vi "Bodies_Init_DH2.vi"(8 "error in (no error)":errorcluster, 10 "KnownDHVars":T3(array[cluster]), 11 "Body.lvclass In":refnum<class "Bodies.lvclass">) -> (0 "error out":errorcluster, 3 "Body.lvclass Out":refnum<class "Bodies.lvclass">)   [LabVIEW 2015, in "Bodies.lvclass"]
uses:
  Bodies.lvclass
  DH_parameters.ctl
  PointOnBody.ctl
  <vilib>/Analysis/Matrix/Datatypes/RealMatrix.ctl
  Bodies.lvclass/Bodies.ctl
  <vilib>/gmath/NI_Gmath.lvlib
  <vilib>/Analysis/Matrix/NI_Matrix.lvlib
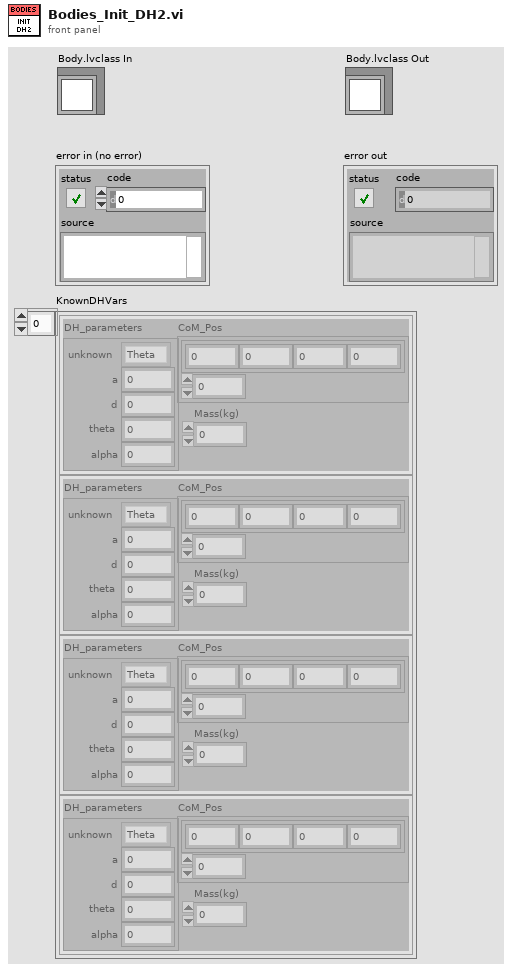
[diagram p1: front panel]
types:
  T1 = typedef "Bodies.lvclass/DH_parameters.ctl" = cluster{"unknown":enum16{"Theta", "Alpha", "a", "d"}, "a":dbl, "d":dbl, "alpha":dbl, "theta":dbl}
  T2 = typedef "Bodies.lvclass/PointOnBody.ctl" = cluster{"Coord4":dbl[], "ID":i32}
  T3 = cluster{"DH_parameters":T1, "CoM_Pos":T2, "Mass(kg)":dbl}[]
  T4 = typedef "NI_Matrix.lvlib/RealMatrix.ctl" = dbl[][]
  T5 = cluster{"Y Values":dbl[][], "Tables":i32[][][], "Variables input decode":i32[], "Variables output decode":i32[]}
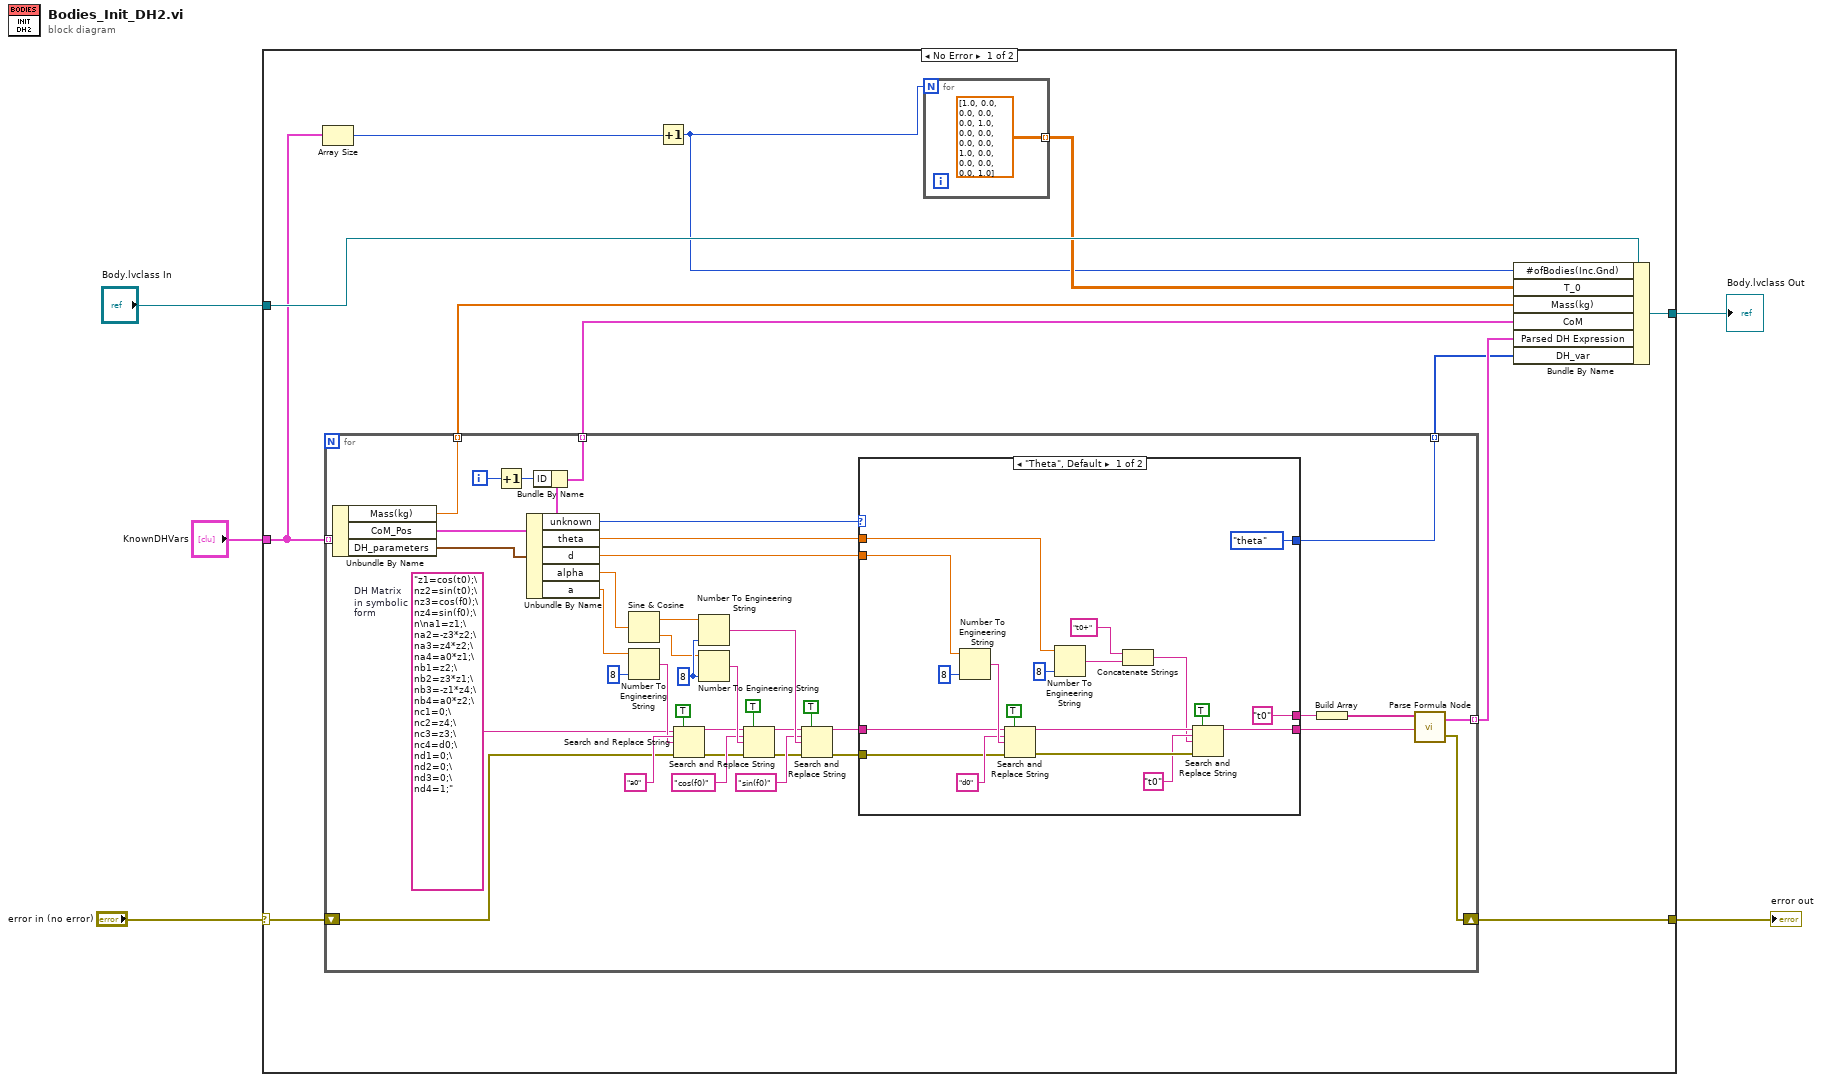
[diagram p0: block diagram]
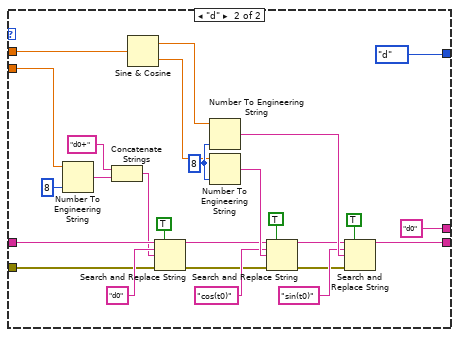
[diagram p2: hidden frame]
diagram:
  n1 = case shown="No Error" "error in (no error)" {
    selector: "error in (no error)" -> [w17 w104]
    tunnel: "KnownDHVars" -> [w11 _]
    tunnel: [w12 w104] -> w5
    tunnel: "Body.lvclass In" -> [w16 w103]
    tunnel: [w14 w103] -> w2
    frame No Error {
      n2 = Array Size(array=w11) -> (size(s)=w10:i32)
      n3 = for {
        tunnel: w11 -> [w55] mode=indexing
        tunnel: [w56] -> w13 mode=indexing
        shift-right: [w57] -> w12
        shift-left: w17 -> [w33]
        tunnel: [w54] -> w8 mode=indexing
        tunnel: [w23] -> w7 mode=indexing
        tunnel: [w20] -> w6 mode=indexing
        i -> [w21]
        w39 = i16 8 ("precision (6)")
        w48 = "z1=cos(t0);\nz2=sin(t0);\nz3=cos(f0);\nz4=sin(f0);\n\na1=z1;\na2=-z3*z2;\na3=z4*z2;\na4=a0*z1;\nb1=z2;\nb2=z3*z1;\nb3=-z1*z4;\nb4=a0*z2;\nc1=0;\nc2=z4;\nc3=z3;\nc4=d0;\nd1=0;\nd2=0;\nd3=0;\nd4=1;"  # DH Matrix in symbolic form
        n4 = Unbundle By Name(w55) -> ("Mass(kg)"=w54:dbl, "CoM_Pos"=w22:T2, "DH_parameters"=w53:T1)
        n5 = Increment(x=w21) -> (x+1=w19:i32)
        n6 = Unbundle By Name(w53) -> ("unknown"=w31:enum16{"Theta", "Alpha", "a", "d"}, "theta"=w30:dbl, "d"=w29:dbl, "alpha"=w36:dbl, "a"=w35:dbl)
        n7 = Bundle By Name(cluster=w22, "ID"=w19) -> (w20:T2)
        n8 = Sine & Cosine(0:w36) -> (1:w37:dbl, 2:w38:dbl)
        n9 = Number To Engineering String(2:i16 8 ("precision (6)"), 4:w35) -> (0:w50:string)  [unwired: 2 in]
        n10 = Search and Replace String(replace all?=TRUE ("replace all? (F)"), input string=w48, search string="a0", replace string=w50, error in=w33) -> (result string=w34:string, error out=w32:errorcluster)  [unwired: 3 in, 2 out]
        n11 = Number To Engineering String(2:w39, 4:w37) -> (0:w46:string)  [unwired: 2 in]
        n12 = Number To Engineering String(2:w39, 4:w38) -> (0:w47:string)  [unwired: 2 in]
        n13 = Search and Replace String(replace all?=TRUE ("replace all? (F)"), input string=w34, search string="cos(f0)", replace string=w47, error in=w32) -> (result string=w42:string, error out=w41:errorcluster)  [unwired: 3 in, 2 out]
        n14 = Search and Replace String(replace all?=TRUE ("replace all? (F)"), input string=w42, search string="sin(f0)", replace string=w46, error in=w41) -> (result string=w28:string, error out=w27:errorcluster)  [unwired: 3 in, 2 out]
        n15 = case shown="\"Theta\", Default" w31 {
          tunnel: w30 -> [w75 w79]
          tunnel: w29 -> [w70 w99]
          tunnel: w28 -> [w69 w98]
          tunnel: w27 -> [w68 w97]
          tunnel: [w60 w78] -> w26
          tunnel: ["t0" ("string") "d0" ("string")] -> w25
          tunnel: [enum16{"theta", "d"}."theta" ("Enum") enum16{"theta", "d"}."d" ("Enum")] -> w23
          frame "Theta", Default {
            n16 = Number To Engineering String(2:i16 8 ("precision (6)"), 4:w70) -> (0:w73:string)  [unwired: 2 in]
            n17 = Search and Replace String(replace all?=TRUE ("replace all? (F)"), input string=w69, search string="d0", replace string=w73, error in=w68) -> (result string=w63:string, error out=w64:errorcluster)  [unwired: 3 in, 2 out]
            n18 = Number To Engineering String(2:i16 8 ("precision (6)"), 4:w75) -> (0:w67:string)  [unwired: 2 in]
            n19 = Concatenate Strings("t0+" ("string"), w67) -> (w61:string)
            n20 = Search and Replace String(replace all?=TRUE ("replace all? (F)"), input string=w63, search string="t0", replace string=w61, error in=w64) -> (result string=w60:string)  [unwired: 3 in, 3 out]
          }
          frame "d" {
            w84 = i16 8 ("precision (6)")
            n21 = Number To Engineering String(2:i16 8 ("precision (6)"), 4:w99) -> (0:w95:string)  [unwired: 2 in]
            n22 = Concatenate Strings("d0+" ("string"), w95) -> (w94:string)
            n23 = Sine & Cosine(0:w79) -> (1:w82:dbl, 2:w83:dbl)
            n24 = Search and Replace String(replace all?=TRUE ("replace all? (F)"), input string=w98, search string="d0", replace string=w94, error in=w97) -> (result string=w81:string, error out=w80:errorcluster)  [unwired: 3 in, 2 out]
            n25 = Number To Engineering String(2:w84, 4:w82) -> (0:w91:string)  [unwired: 2 in]
            n26 = Number To Engineering String(2:w84, 4:w83) -> (0:w92:string)  [unwired: 2 in]
            n27 = Search and Replace String(replace all?=TRUE ("replace all? (F)"), input string=w81, search string="cos(t0)", replace string=w92, error in=w80) -> (result string=w87:string, error out=w86:errorcluster)  [unwired: 3 in, 2 out]
            n28 = Search and Replace String(replace all?=TRUE ("replace all? (F)"), input string=w87, search string="sin(t0)", replace string=w91, error in=w86) -> (result string=w78:string)  [unwired: 3 in, 3 out]
          }
        }
        n29 = Build Array(w25) -> (w24:string[])
        n30 = call <vilib>:"Parse Formula Node.vi"("formula"=w26, "Variables Input"=w24) -> ("error out"=w57:errorcluster, "Parsed Formula Node"=w56:T5)  [unwired: 2 in]
      }
      n31 = Increment(x=w10) -> (x+1=w9:i32)
      n32 = for {
        N: w9 -> [_]
        tunnel: [T4 [[1.0, 0.0, 0.0, 0.0], [0.0, 1.0, 0.0, 0.0], [0.0, 0.0, 1.0, 0.0], [0.0, 0.0, 0.0, 1.0]] ("Real Matrix")] -> w15 mode=indexing
      }
      n33 = Bundle By Name(cluster=w16, "#ofBodies(Inc.Gnd)"=w9, "T_0"=w15, "Mass(kg)"=w8, "CoM"=w6, "Parsed DH Expression"=w13, "DH_var"=w7) -> (w14:refnum<class "Bodies.lvclass">)
    }
    frame Error {
    }
  }
  "error out" <- w5
  "Body.lvclass Out" <- w2
